vi "AssertFloatingPoint_Anything.vi"(8 "error in":errorcluster, 11 "Anything":refnum<class "Anything.lvclass">) -> (0 "error out":errorcluster, 3 "Anything":refnum<class "Anything.lvclass">)   [LabVIEW 2020, in "OpenLvVision_OpenCv.lvlib"]
uses:
  OpenLvVision_OpenCv.lvlib
  Anything.lvclass
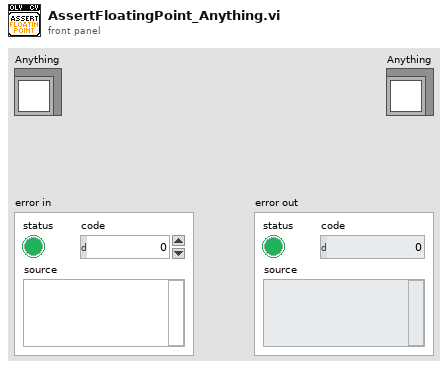
[diagram p1: front panel]
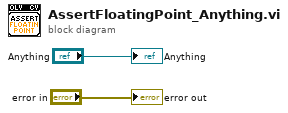
[diagram p0: block diagram]
diagram:
  "error out" <- "error in"
  "Anything" <- "Anything"
